vi "Temperature Guard.vi"(8 "error in (no error)":errorcluster, 11 "Freezer in":refnum<class "Freezer.lvclass">) -> (0 "error out":errorcluster, 1 "Low Temp":dbl, 2 "Low Temp reached":bool, 3 "Freezer in 2":refnum<class "Freezer.lvclass">, 4 "Current Temp":dbl, 5 "s? t:f 2":cluster{dbl, "Syringe TC":dbl, "Lower":dbl})   [LabVIEW 2015, in "cRIO-Carbondioxide.lvlib" / "CO2-Actor.lvlib" / "Freezer.lvclass"]
uses:
  Freezer.lvclass
  Freezer.lvclass/Freezer.ctl
  <vilib>/ptbypt/NI_PtbyPt.lvlib
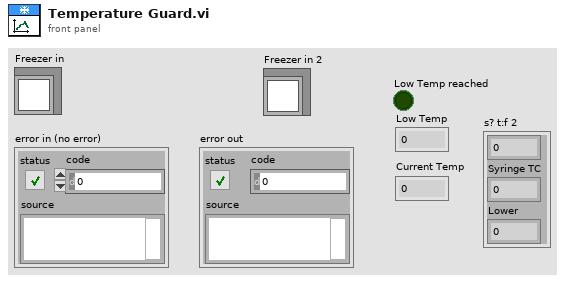
[diagram p1: front panel]
types:
  T1 = enum32{"Invalid", "Standard", "Closed", "Hidden", "Minimized", "Maximized"}
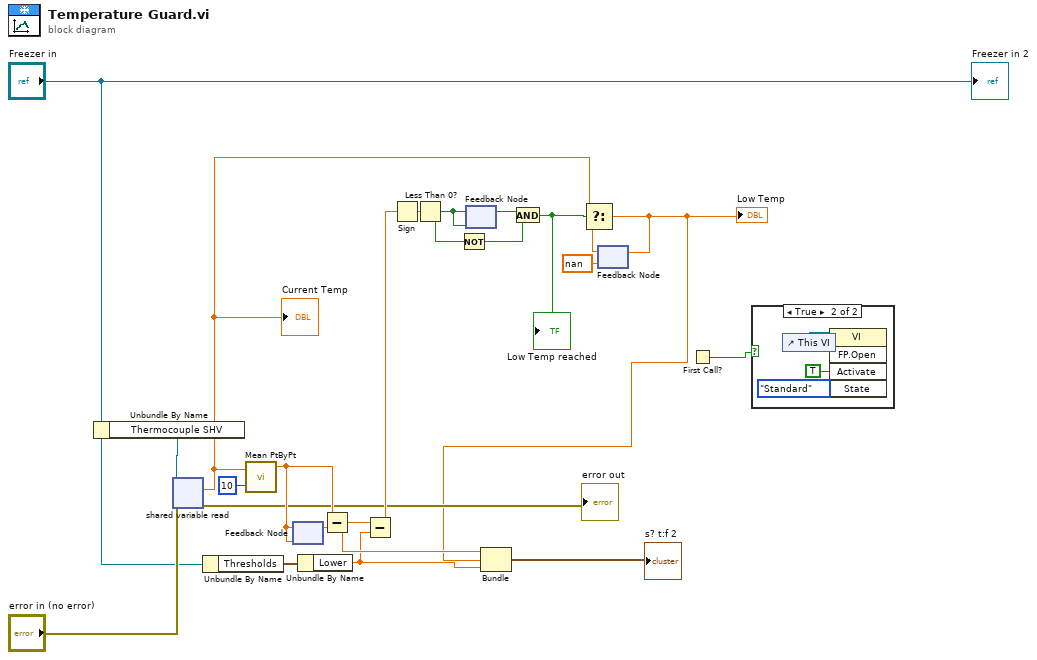
[diagram p0: block diagram]
diagram:
  n1 = Unbundle By Name("Freezer in") -> ("Thermocouple SHV"=w18:refnum<k21>)
  n2 = shared-variable-read(w18, "error in (no error)") -> (→"error out":errorcluster, w8:dbl)  [unwired: 2 out]
  "Current Temp" <- w8
  n3 = Unbundle By Name("Freezer in") -> ("Thresholds"=w20:cluster{"Upper":dbl, "Lower":dbl})
  n4 = call <vilib>:"Mean PtByPt.vi"("x"=w8, "sample length"=10) -> ("mean"=w22:dbl)  [unwired: 2 in, 1 out]
  n5 = feedback #1(w22) -> (w21:dbl)
  n6 = feedback-in #1(w22) -> ()
  n7 = Unbundle By Name(w20) -> ("Lower"=w5:dbl)
  n8 = Subtract(x=w22, y=w21) -> (x-y=w13:dbl)
  n9 = Subtract(x=w13, y=w5) -> (x-y=w16:dbl)
  n10 = Sign(1:w16) -> (0:w15:dbl)
  n11 = Less Than 0?(x=w15) -> (x < 0?=w12:bool)
  n12 = Not(x=w12) -> (.not. x?=w11:bool)
  n13 = feedback-in #2(w12) -> ()
  n14 = feedback #2(w12) -> (w14:bool)
  n15 = And(x=w14, y=w11) -> (x .and. y?=w9:bool)
  "Low Temp reached" <- w9
  n16 = feedback #3(nan ("Syringe TC")) -> (w7:dbl)
  n17 = Select(t=w8, s=w9, f=w7) -> (s? t:f=w2:dbl)
  "Low Temp" <- w2
  n18 = Bundle(w13, "Syringe TC"=w2, "Lower"=w5) -> (→"s? t:f 2":cluster{dbl, "Syringe TC":dbl, "Lower":dbl})  [unwired: 1 in]
  n19 = feedback-in #3(w2) -> ()
  n20 = First Call?() -> (First Call?: T/F=w4:bool)
  n21 = case shown="True" w4 {
    frame False {
    }
    frame True {
      n22 = control-ref of="This VI"() -> (w25:refnum<vi>)
      n23 = invoke class="VI" method="FP.Open"(reference=w25, "Activate"=TRUE ("Activate?"), "State"=T1."Standard") -> ()  [unwired: 2 in, 5 out]
    }
  }
  "Freezer in 2" <- "Freezer in"
